vi "GetDirectory.vi"(11 "tracpoint directories":T1) -> (2 "tracepoint directory":path, 3 "log directory":path)   [LabVIEW 2017, in "TraceLogger.lvlib"]
uses:
  <vilib>/addons/TraceLogger/TraceLogger.lvlib
  <vilib>/addons/TraceLogger/controls/TracpointDirectories.ctl
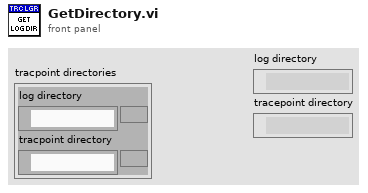
[diagram p1: front panel]
types:
  T1 = typedef "TracpointDirectories.ctl" = cluster{"log directory":path, "tracpoint directory":path}
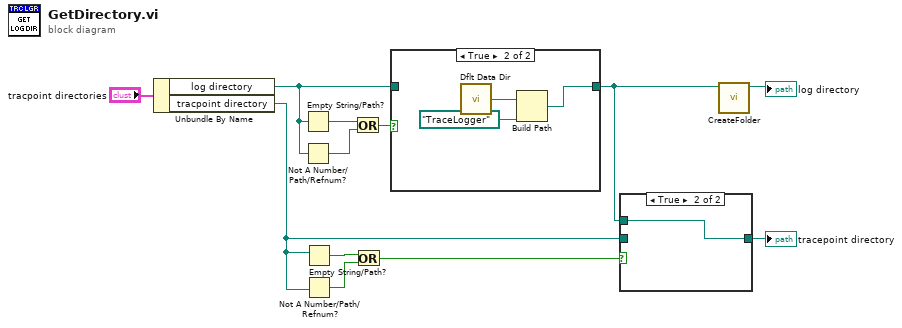
[diagram p0: block diagram]
diagram:
  n1 = Unbundle By Name("tracpoint directories") -> ("log directory"=w7:path, "tracpoint directory"=w2:path)
  n2 = Empty String/Path?(string/path=w7) -> (empty?=w12:bool)
  n3 = Not A Number/Path/Refnum?(number/path/refnum=w7) -> (NaN/Path/Refnum?=w11:bool)
  n4 = Empty String/Path?(string/path=w2) -> (empty?=w5:bool)
  n5 = Not A Number/Path/Refnum?(number/path/refnum=w2) -> (NaN/Path/Refnum?=w6:bool)
  n6 = Or(x=w12, y=w11) -> (x .or. y?=w10:bool)
  n7 = Or(x=w5, y=w6) -> (x .or. y?=w4:bool)
  n8 = case shown="True" w10 {
    tunnel: [w13 w14] -> w3
    tunnel: w7 -> [w13 _]
    frame False {
    }
    frame True {
      n9 = call <vilib>:"Dflt Data Dir.vi"() -> ("App:Default Data Directory"=w16:path)
      n10 = Build Path(base path=w16, name or relative path=path "TraceLogger" ("system directory")) -> (appended path=w14:path)
    }
  }
  n11 = case shown="True" w4 {
    tunnel: w3 -> [_ w18]
    tunnel: [w17 w18] -> w1
    tunnel: w2 -> [w17 _]
    frame False {
    }
    frame True {
    }
  }
  "tracepoint directory" <- w1
  n12 = call <vilib>:"CreateFolder.vi"("folder"=w3) -> ("folder out"=→"log directory":path)  [unwired: 9 in, 1 out]
